vi "standBy.vi"(8 "error in (no error)":errorcluster, 11 "Context in":refnum<class "Context.lvclass">) -> (0 "error out":errorcluster, 3 "Context out":refnum<class "Context.lvclass">)   [LabVIEW 2013, in "Context.lvclass"]
uses:
  Context.lvclass
  Context.lvclass/Context.ctl
  State/State.lvclass
  Model/Model/Model/Model.lvclass
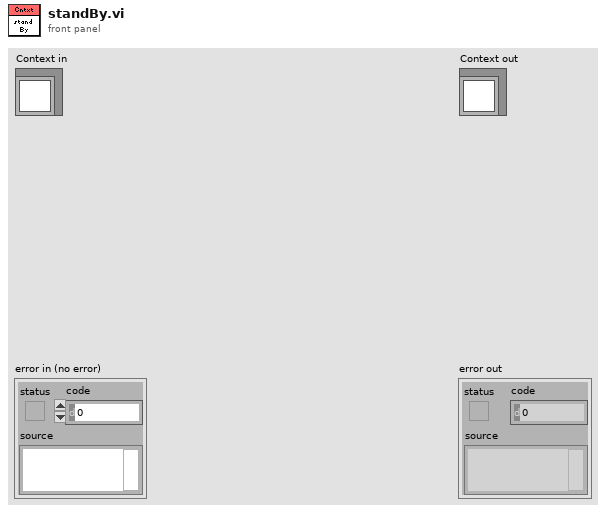
[diagram p1: front panel]
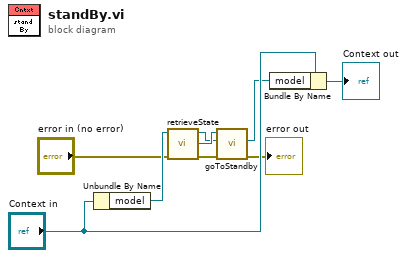
[diagram p0: block diagram]
diagram:
  n1 = Unbundle By Name("Context in") -> ("model"=w8:refnum<class "Model.lvclass">)
  n2 = call "retrieveState.vi"("error in (no error)"="error in (no error)", "Model in"=w8) -> ("error out"=w1:errorcluster, "state"=w9:refnum<class "State.lvclass">, "Model out"=w7:refnum<class "Model.lvclass">)  [unwired: 7 in]
  n3 = call-dynamic "goToStandby.vi"("error in (no error)"=w1, "model"=w7, "State in"=w9) -> ("error out"=→"error out":errorcluster, "model 2"=w4:refnum<class "Model.lvclass">)  [unwired: 6 in, 1 out]
  n4 = Bundle By Name(cluster="Context in", "model"=w4) -> (→"Context out":refnum<class "Context.lvclass">)
